vi "Exemple_Preprocessing_FunctionTransformer.vi"() -> ()   [LabVIEW 2020]
uses:
  Objet/6 - Datasets Transformation/6.3 - Processing Data/FunctionTransformer/FunctionTransformer.lvclass
panel:
  in  "y":string[][](array[string])
  in  "X":string[][](array[string])=[["0", "1"], ["2", "3"]]
  out "Data":T1
  out "error out":errorcluster
  in  "error in":errorcluster caption="entrée d'erreur"
  in  "FunctionTransformer":T2={"func_callable"="np.log1p", "inverse_func_callable"="None", "validate"=FALSE, "accept_sparse"=FALSE, "check_inverse"=TRUE, "kw_args"={"key"=[], "Value"=[]}, "inv_kw_args"={"key"=[], "Value"=[]}}
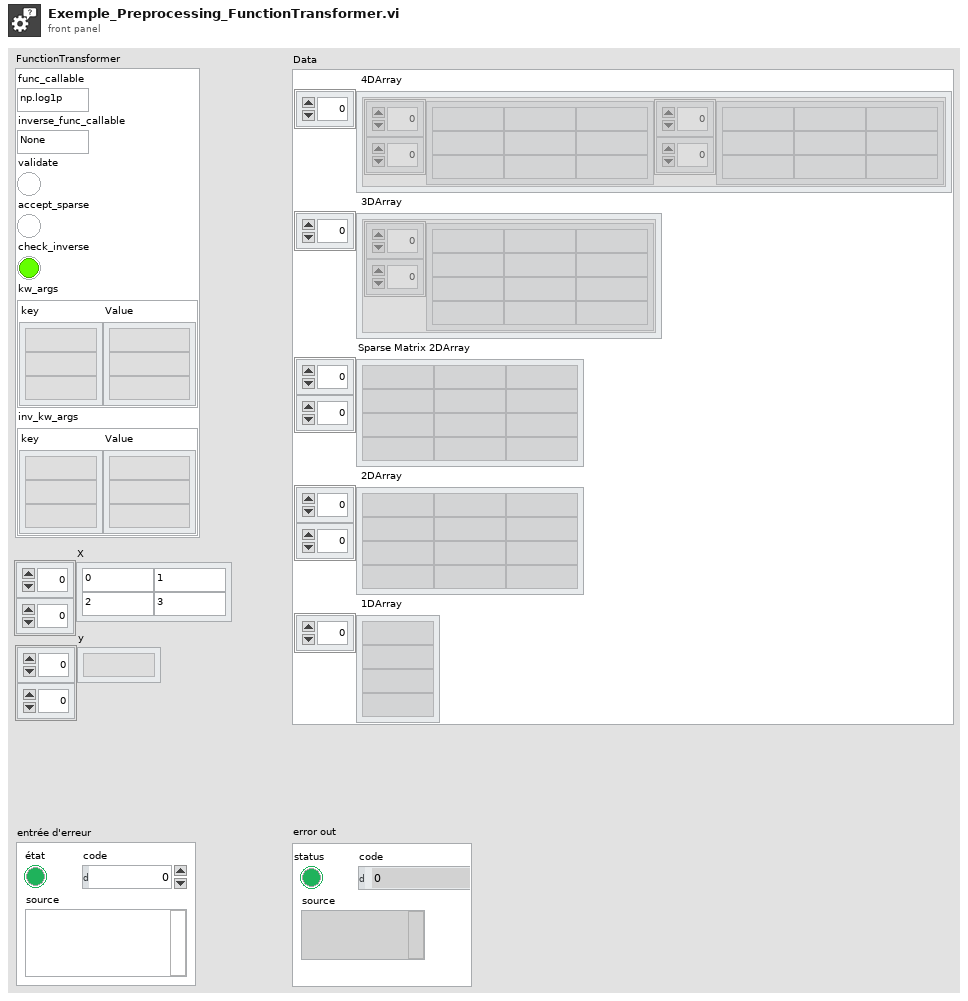
[diagram p1: front panel]
types:
  T1 = cluster{" 4DArray":cluster{"1":string[][], "2":string[][]}[], " 3DArray":cluster{"Tableau":string[][]}[], "Sparse Matrix 2DArray":string[][], " 2DArray":string[][], " 1DArray":string[]}
  T2 = cluster{"func_callable":string, "inverse_func_callable":string, "validate":bool, "accept_sparse":bool, "check_inverse":bool, "kw_args":cluster{"key":string[], "Value":string[]}, "inv_kw_args":cluster{"key":string[], "Value":string[]}}
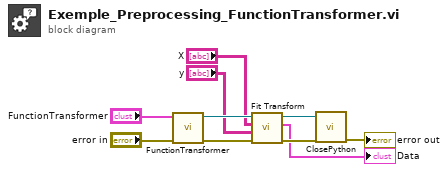
[diagram p0: block diagram]
diagram:
  n1 = call "FunctionTransformer.vi"("error in (no error)"="error in", "FunctionTransformer"="FunctionTransformer") -> ("error out"=w5:errorcluster, "FunctionTransformer.lvclass"=w8:refnum<class "FunctionTransformer.lvclass">)  [unwired: 8 in]
  n2 = call-dynamic "Fit Transform.vi"("error in (no error)"=w5, "y"="y", "X"="X", "FunctionTransformer.lvclass"=w8) -> ("error in (no error)"=w3:errorcluster, "Data"=→"Data":T1, "FunctionTransformer.lvclass"=w4:refnum<class "FunctionTransformer.lvclass">)  [unwired: 5 in]
  n3 = call-dynamic "ClosePython.vi"("error in (no error)"=w3, "Scikit-learn en entrée"=w4) -> ("error out"=→"error out":errorcluster)  [unwired: 8 in, 1 out]
